vi "Joysticks Config.vi"(9 "Secondary Controller USB Output":T1, 11 "Primary Controller Usb Output":T1) -> ()   [LabVIEW 2012]
uses:
  <vilib>/Rock Robotics/WPI/Joystick/WPI_JoystickDeviceEnum.ctl
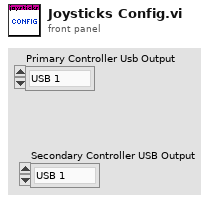
[diagram p1: front panel]
types:
  T1 = typedef "WPI_JoystickDeviceEnum.ctl" = enum16{"USB 1", "USB 2", "USB 3", "USB 4", "Kinect 1", "Kinect 2"}
  T2 = typedef "WPI_JoystickDevRef.ctl" = cluster{"Device":T1}
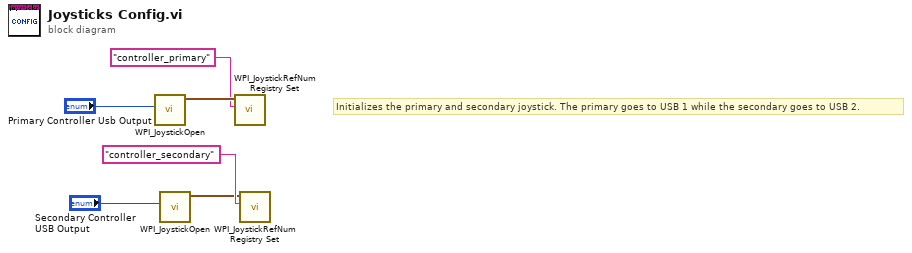
[diagram p0: block diagram]
diagram:
  # "Initializes the primary and secondary joystick. The primary goes to USB 1 while the secondary goes to USB 2."
  n1 = call <vilib>:"WPI_JoystickOpen.vi"("JoystickDevice"="Primary Controller Usb Output") -> ("JoystickDevRef"=w6:T2)  [unwired: 10 in]
  n2 = call <vilib>:"WPI_JoystickOpen.vi"("JoystickDevice"="Secondary Controller USB Output") -> ("JoystickDevRef"=w1:T2)  [unwired: 10 in]
  n3 = call <vilib>:"WPI_JoystickRefNum Registry Set.vi"("refnum name"="controller_primary", "JoystickDevRef"=w6) -> ()  [unwired: 8 in, 2 out]
  n4 = call <vilib>:"WPI_JoystickRefNum Registry Set.vi"("refnum name"="controller_secondary", "JoystickDevRef"=w1) -> ()  [unwired: 8 in, 2 out]
